vi "TCS_Tx_VISA.vi"() -> ()   [LabVIEW 2018]
uses:
  RxTx/RxTx.lvclass
  Serial Communication/Serial Communication.lvclass
panel:
  in  "Serial Communication in":refnum<class "Serial Communication.lvclass">
  in  "RxTx.lvclass":refnum<class "RxTx.lvclass">
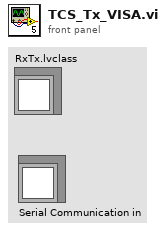
[diagram p1: front panel]
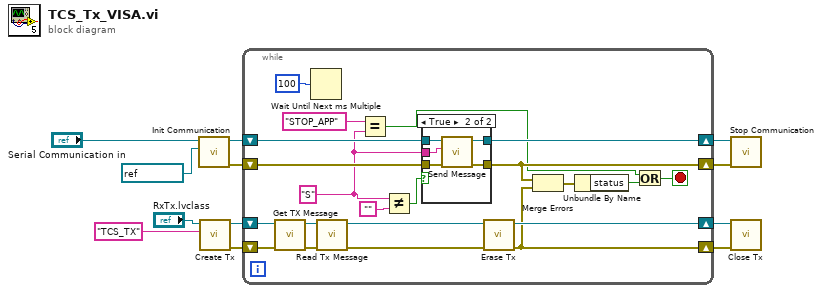
[diagram p0: block diagram]
diagram:
  n1 = call "Init Communication.vi"("VISA resource name"=refnum<visa-resource-name> "COM2", "Serial Communication in"="Serial Communication in") -> ("error out"=w3:errorcluster, "Serial Communication out"=w4:refnum<class "Serial Communication.lvclass">)  [unwired: 8 in]
  n2 = call "Create Tx.vi"("Writer Name"="TCS_TX" ("Reader Name"), "RxTx in"="RxTx.lvclass") -> ("error out"=w11:errorcluster, "RxTx out"=w12:refnum<class "RxTx.lvclass">)  [unwired: 8 in]
  n3 = while {
    shift-right: [w25] -> w5
    shift-left: w3 -> [w27]
    shift-right: [w26] -> w6
    shift-left: w4 -> [w28]
    shift-right: [w20] -> w8
    shift-left: w11 -> [w29]
    shift-right: [w22] -> w9
    shift-left: w12 -> [w30]
    stop <- w17 stop-if-true
    w13 = "S" ("y")
    n4 = call "Get TX Message.vi"("error in (no error)"=w29, "RxTx in"=w30) -> ("error out"=w32:errorcluster, "RxTx out"=w31:refnum<class "RxTx.lvclass">)  [unwired: 8 in]
    n5 = Wait Until Next ms Multiple(millisecond multiple=u32 100 ("milliseconds to wait")) -> ()  [unwired: 1 out]
    n6 = call "Read Tx Message.vi"("error in (no error)"=w32, "RxTx in"=w31) -> ("error out"=w21:errorcluster, "RxTx out"=w23:refnum<class "RxTx.lvclass">)  [unwired: 7 in, 1 out]
    n7 = Equal?(x="STOP_APP", y=w13) -> (x = y?=w19:bool)
    n8 = Not Equal?(x=w13, y="") -> (x != y?=w15:bool)
    n9 = case shown="True" w15 {
      tunnel: w28 -> [w35 w36]
      tunnel: w27 -> [w34 w39]
      tunnel: [w35 w37] -> w26
      tunnel: w13 -> [_ w40]
      tunnel: [w34 w38] -> w25
      frame False {
      }
      frame True {
        n10 = call "Send Message.vi"("error in (no error)"=w39, "Message"=w40, "Serial Communication in"=w36) -> ("error out"=w38:errorcluster, "Serial Communication out"=w37:refnum<class "Serial Communication.lvclass">)  [unwired: 7 in]
      }
    }
    n11 = call "Erase Tx.vi"("error in (no error)"=w21, "RxTx in"=w23) -> ("error out"=w20:errorcluster, "RxTx out"=w22:refnum<class "RxTx.lvclass">)  [unwired: 8 in]
    n12 = Merge Errors(w25, w20) -> (w33:errorcluster)
    n13 = Unbundle By Name(w33) -> ("status"=w18:bool)
    n14 = Or(x=w19, y=w18) -> (x .or. y?=w17:bool)
  }
  n15 = call "Stop Communication.vi"("error in (no error)"=w5, "Serial Communication in"=w6) -> ()  [unwired: 8 in, 2 out]
  n16 = call "Close Tx.vi"("error in (no error)"=w8, "RxTx in"=w9) -> ()  [unwired: 8 in, 2 out]
